vi "DataLog Read Recovery File.vi"(11 "error in (no error)":errorcluster) -> (8 "aggregation entries":T1[](array[typedef]) {"point"."value" format="%.3e"; "point"."time" format="%<%H:%M:%S%2u\n%Y/%m/%d>T"}, 15 "error out":errorcluster)   [LabVIEW 2012]
doc: "Read the recovery file that reflects the aggregation buffer back from disk."
uses:
  typedefs/clusters/t_DataLog Aggregation Entry.ctl
  typedefs/clusters/t_DataLog Point.ctl
  glb_DataLog Runtime Parameterisation.vi
  glb_DataLog MCVD.vi
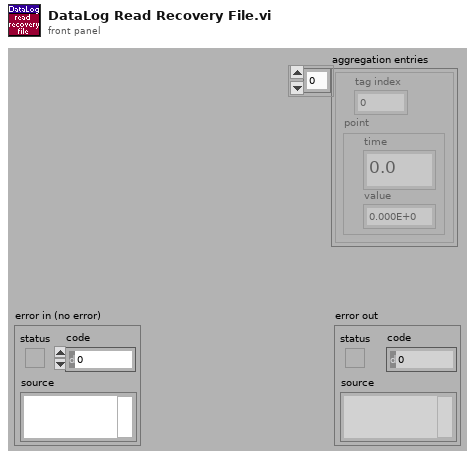
[diagram p1: front panel]
types:
  T1 = typedef "t_DataLog Aggregation Entry.ctl" = cluster{"tag index":i32, "point":T2}
  T2 = typedef "t_DataLog Point.ctl" = cluster{"time":dbl, "value":dbl}
  T3 = enum16{"deny read/write", "deny write-only", "deny none"}
  T4 = enum16{"read/write", "read-only", "write-only", "write-only (truncate)"}
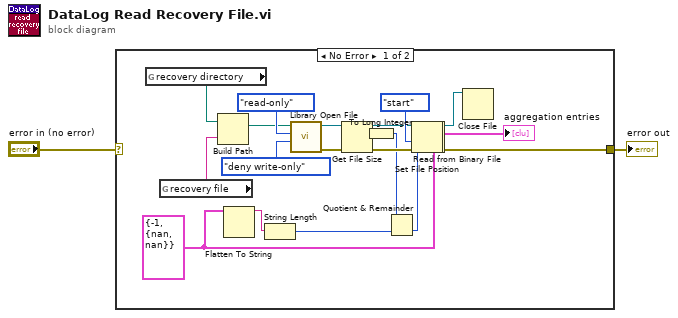
[diagram p0: block diagram]
diagram:
  n1 = case shown="No Error" "error in (no error)" {
    selector: "error in (no error)" -> [_ w24]
    tunnel: [w7 w24] -> w2
    frame No Error {
      w16 = T1 {"tag index"=-1, "point"={"time"=nan, "value"=nan}} ("aggregation entry")
      n2 = global read "glb_DataLog Runtime Parameterisation.vi" "recovery directory"() -> (w6:path)
      n3 = global read "glb_DataLog MCVD.vi" "recovery file"() -> (w23:string)
      n4 = Build Path(base path=w6, name or relative path=w23) -> (appended path=w13:path)
      n5 = Flatten To String(anything=w16) -> (data string=w19:string)  [unwired: 3 in, 2 out]
      n6 = String Length(string=w19) -> (length=w20:i32)
      n7 = call "Library Open File.vi"("deny mode (deny none)"=T3."deny write-only" ("deny mode (2)"), "open mode (read/write)"=T4."read-only" ("open mode (0)"), "file path"=w13) -> ("error out"=w12:errorcluster, "refnum"=w11:refnum<file>)  [unwired: 3 in]
      n8 = Get File Size(file=w11, error in=w12) -> (refnum out=w9:refnum<file>, size (in bytes)=w5:i64, 0:w10:errorcluster)
      n9 = To Long Integer(number=w5) -> (32bit integer=w8:i32)
      n10 = Quotient & Remainder(x=w8, y=w20) -> (floor(x/y)=w18:i32)  [unwired: 1 out]
      n11 = Set File Position(refnum=w9, from (0:start)=enum16{"start", "end", "current"}."start" ("pos mode (0:2)"), error in=w10) -> (refnum out=w4:refnum<file>, error out=w3:errorcluster)  [unwired: 1 in]
      n12 = Read from Binary File(5:w16, 8:w3, 10:w18, 11:w4) -> (0:w7:errorcluster, 2:→"aggregation entries":T1[], 3:w15:refnum<file>)  [unwired: 2 in, 1 out]
      n13 = Close File(refnum=w15) -> ()  [unwired: 1 in, 2 out]
    }
    frame Error {
    }
  }
  "error out" <- w2
